vi "CgLight.vi"(3 "error in (no error)":errorcluster, 4 "Flashes":i32=1, 5 "Mode":enum16{"Off", "On", "Flash"}(ring), 6 "VISA resource name":refnum<visa-resource-name>) -> (0 "error out":errorcluster, 2 "VISA resource name out":refnum<visa-resource-name>)   [LabVIEW 2012]
doc: "Allows control of the light on the cyberglove. Can set the light to \"on\" \"off\" or \"flash\". \"Flash\" causes the light to flash (on for 100ms, off for 100ms) the number of times given by the flashes input (default, 1)."
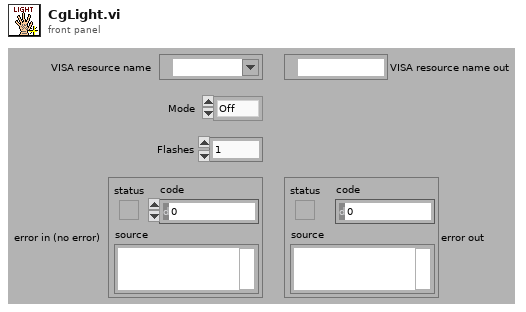
[diagram p1: front panel]
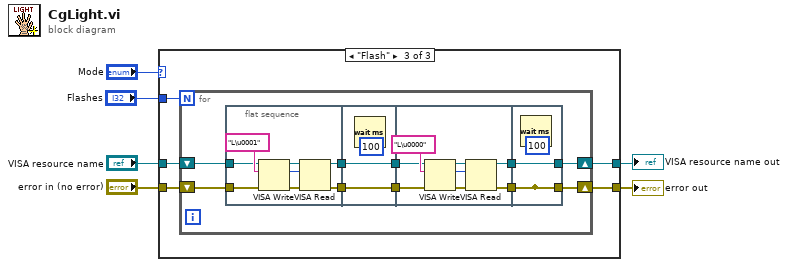
[diagram p0: block diagram]
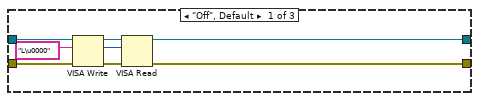
[diagram p2: hidden frame]
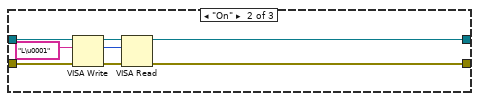
[diagram p3: hidden frame]
diagram:
  n1 = case shown="\"Flash\"" "Mode" {
    tunnel: "VISA resource name" -> [w13 w21 w27]
    tunnel: "error in (no error)" -> [w14 w22 w26]
    tunnel: [w8 w16 w25] -> w2
    tunnel: [w7 w15 w24] -> w1
    tunnel: "Flashes" -> [_ _ w23]
    frame "Off", Default {
      n2 = VISA Write(VISA resource name=w13, write buffer="L\u0000", error in (no error)=w14) -> (VISA resource name out=w9:refnum<visa-resource-name>, return count=w10:u32, error out=w11:errorcluster)
      n3 = VISA Read(VISA resource name=w9, byte count=w10, error in (no error)=w11) -> (VISA resource name out=w8:refnum<visa-resource-name>, error out=w7:errorcluster)  [unwired: 2 out]
    }
    frame "On" {
      n4 = VISA Write(VISA resource name=w21, write buffer="L\u0001", error in (no error)=w22) -> (VISA resource name out=w17:refnum<visa-resource-name>, return count=w18:u32, error out=w19:errorcluster)
      n5 = VISA Read(VISA resource name=w17, byte count=w18, error in (no error)=w19) -> (VISA resource name out=w16:refnum<visa-resource-name>, error out=w15:errorcluster)  [unwired: 2 out]
    }
    frame "Flash" {
      n6 = for {
        N: w23 -> [_]
        shift-right: [w29] -> w25
        shift-left: w27 -> [w37]
        shift-right: [w28] -> w24
        shift-left: w26 -> [w36]
        n7 = flat-sequence {
          tunnel: w37 -> [w41]
          tunnel: w36 -> [w40]
          tunnel: [w39] -> w34
          tunnel: [w38] -> w32
          tunnel: [w47] -> w35
          tunnel: w34 -> [w47]
          tunnel: [w46] -> w33
          tunnel: w32 -> [w46]
          tunnel: w35 -> [w52]
          tunnel: w33 -> [w51]
          tunnel: [w50] -> w31
          tunnel: [w49] -> w30
          tunnel: w31 -> [w58]
          tunnel: [w57] -> _
          tunnel: w30 -> [w57]
          tunnel: [w58] -> w29
          tunnel: [w57] -> w28
          frame #0 {
            n8 = VISA Write(VISA resource name=w41, write buffer="L\u0001", error in (no error)=w40) -> (VISA resource name out=w44:refnum<visa-resource-name>, return count=w43:u32, error out=w42:errorcluster)
            n9 = VISA Read(VISA resource name=w44, byte count=w43, error in (no error)=w42) -> (VISA resource name out=w39:refnum<visa-resource-name>, error out=w38:errorcluster)  [unwired: 2 out]
          }
          frame #1 {
            n10 = Wait (ms)(milliseconds to wait=u32 100) -> ()  [unwired: 1 out]
          }
          frame #2 {
            n11 = VISA Write(VISA resource name=w52, write buffer="L\u0000", error in (no error)=w51) -> (VISA resource name out=w55:refnum<visa-resource-name>, return count=w54:u32, error out=w53:errorcluster)
            n12 = VISA Read(VISA resource name=w55, byte count=w54, error in (no error)=w53) -> (VISA resource name out=w50:refnum<visa-resource-name>, error out=w49:errorcluster)  [unwired: 2 out]
          }
          frame #3 {
            n13 = Wait (ms)(milliseconds to wait=u32 100) -> ()  [unwired: 1 out]
          }
        }
      }
    }
  }
  "VISA resource name out" <- w2
  "error out" <- w1
